vi "initialized butterworth.vi"(6 "pre-buffer size":i32=10000, 8 "low cutoff freq: fl":dbl=0.12500000000000006 format="%0.4f", 9 "high cutoff freq: fh":dbl=0.45000000000000007 format="%0.2f", 10 "sampling freq: fs":dbl=1.0 format="%0.2f", 11 "Waveform":waveform(dbl)) -> (3 "Filtered Waveform":waveform(dbl))   [LabVIEW 2012]
uses:
  <vilib>/Analysis/3filter.llb/Butterworth Filter (DBL).vi
  <vilib>/Analysis/NI_AALBase.lvlib
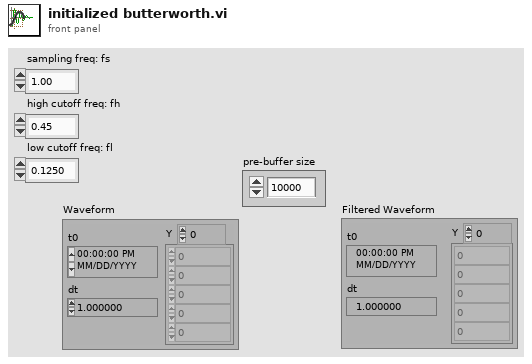
[diagram p1: front panel]
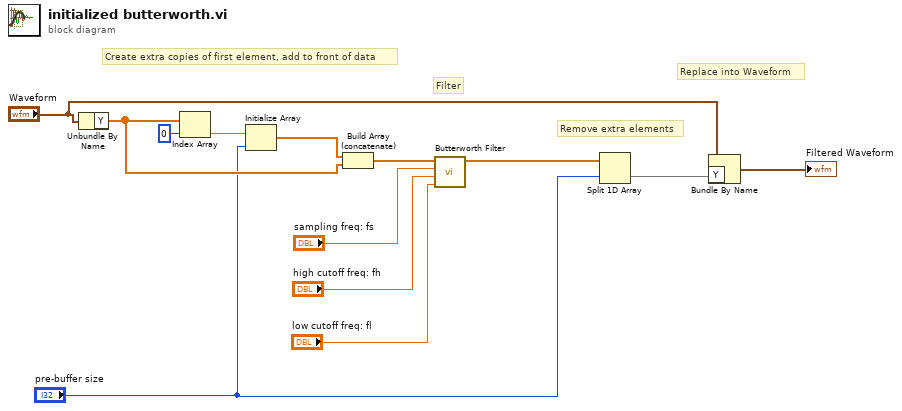
[diagram p0: block diagram]
diagram:
  # "Replace into Waveform"
  # "Remove extra elements"
  # "Filter"
  # "Create extra copies of first element, add to front of data"
  n1 = Unbundle By Name("Waveform") -> ("Y"=w11:dbl[])
  n2 = Index Array(array=w11, index=0) -> (element=w13:dbl)
  n3 = Initialize Array(w13, "pre-buffer size") -> (w12:dbl[])
  n4 = Build Array (concatenate)(w12, w11) -> (w5:dbl[])
  n5 = call-poly <vilib>:"Butterworth Filter.vi"("low cutoff freq: fl"="low cutoff freq: fl", "high cutoff freq: fh"="high cutoff freq: fh", "sampling freq: fs"="sampling freq: fs", "X"=w5) -> ("Filtered X"=w7:dbl[])  [unwired: 4 in, 1 out]
  n6 = Split 1D Array(array=w7, index="pre-buffer size") -> (second subarray=w4:dbl[])  [unwired: 1 out]
  n7 = Bundle By Name(cluster="Waveform", "Y"=w4) -> (→"Filtered Waveform":waveform(dbl))
